vi "Menu Handler.vi"(7 "Sub Panel":refnum<vi>, 8 "error in (no error)":errorcluster, 9 "ItemTag":string, 10 "Menu in":refnum<k9>, 11 "queue out":refnum<queue>) -> (0 "Error Out":errorcluster, 3 "Log 10?":bool=TRUE)   [LabVIEW 2015]
uses:
  Type Defs/OCT Hardware States.ctl
  Classes/DAQ/DAQ Status States.ctl
  Classes/DAQ/DAQ Control Functional Global States.ctl
  Classes/Processing/Filter/Filter List.ctl
  Classes/Processing/Filter/Kernel Size.ctl
  Classes/Processing/Processing.lvclass
  Classes/Processing/Intensity/Intensity Processing.lvclass
  Classes/Processing/Filter/Filter.lvclass
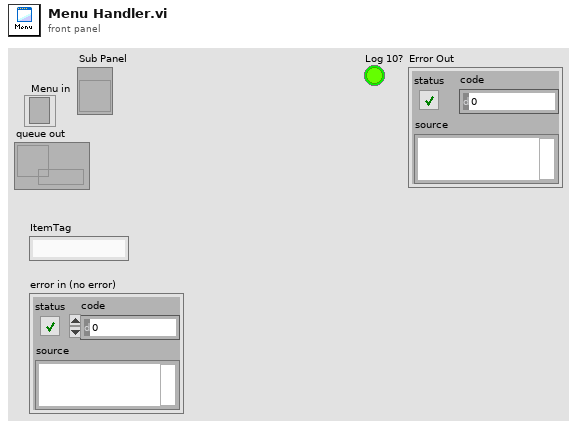
[diagram p1: front panel]
types:
  T1 = typedef "DAQ Status States.ctl" = enum16{"Get", "Show"}
  T2 = typedef "OCT Hardware States.ctl" = enum16{"Acquire Data", "Initialize Laser", "Initialize Galvos", "Startup", "Reset DAQ", "Background Subtraction", "Acquire Background", "Update DAQ Parameters", "Stop", "Set Clock", "Initialize DAQ", "Set Resampling Array", "Save Sweep", "Configure Laser", "128 x 128", "512 x 1", "512 x 512", "Review Data", "Configure Trigger", "Update Galvos", "Update Filter", "Fire Digital Output", "Configure Digital Output", "Save Galvo Settings", "Load Galvo Settings"}
  T3 = typedef "DAQ Control Functional Global States.ctl" = enum16{"Status", "Set Processing Finished", "Reset", "Clear", "Set DAQ Finished"}
  T4 = enum32{"Invalid", "Standard", "Closed", "Hidden", "Minimized", "Maximized"}
  T5 = typedef "Kernel Size.ctl" = enum16{"3x3", "5x5", "3x5", "5x3"}
  T6 = typedef "Filter.lvclass/Filter List.ctl" = enum16{"None", "Std. Dev.", "Speckle Variance"}
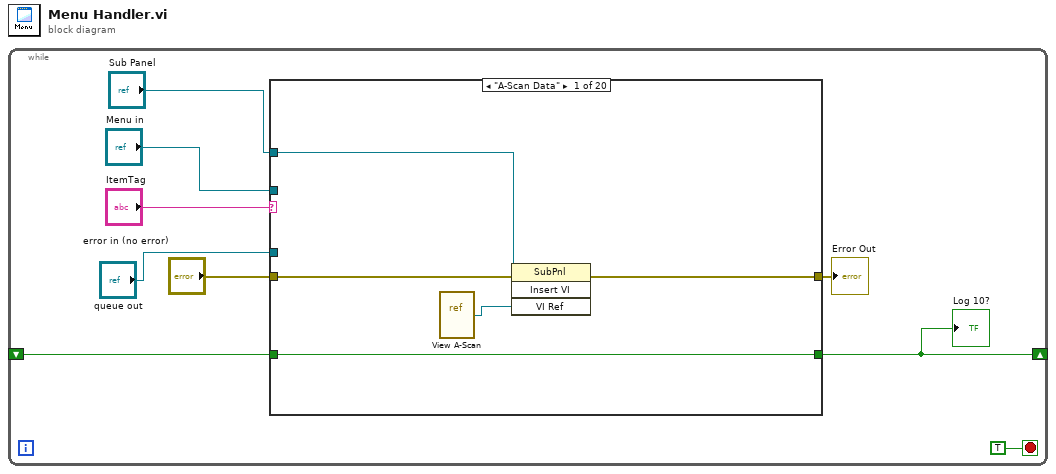
[diagram p0: block diagram]
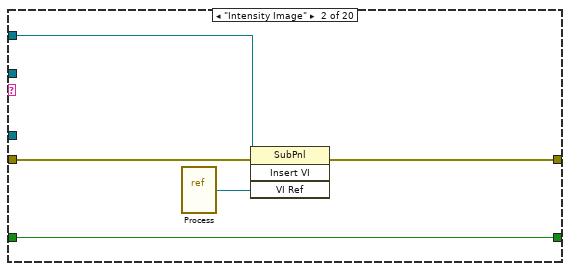
[diagram p2: hidden frame]
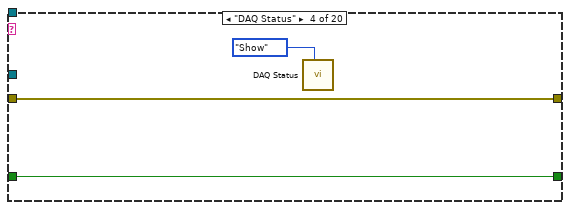
[diagram p4: hidden frame]
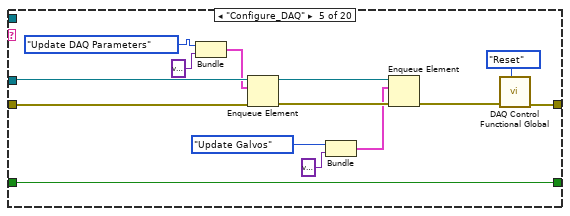
[diagram p5: hidden frame]
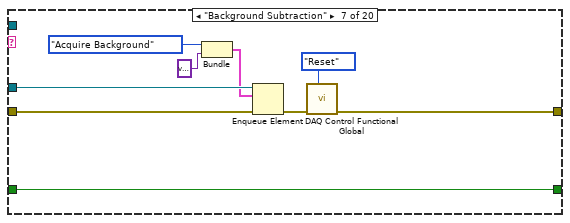
[diagram p7: hidden frame]
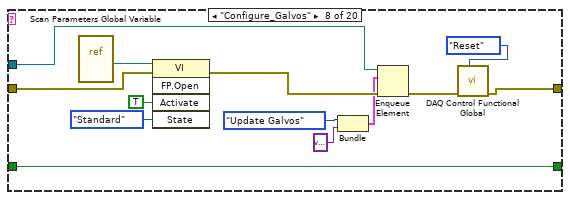
[diagram p8: hidden frame]
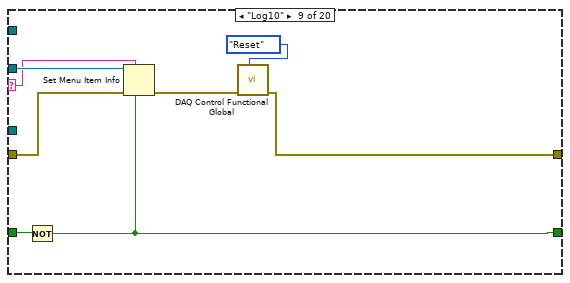
[diagram p9: hidden frame]
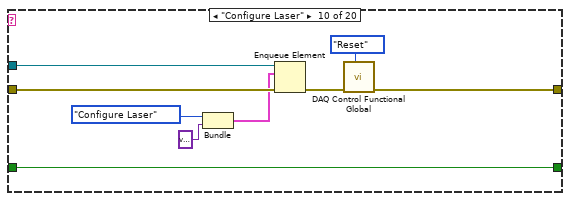
[diagram p10: hidden frame]
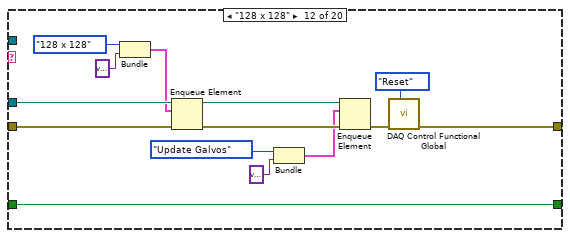
[diagram p12: hidden frame]
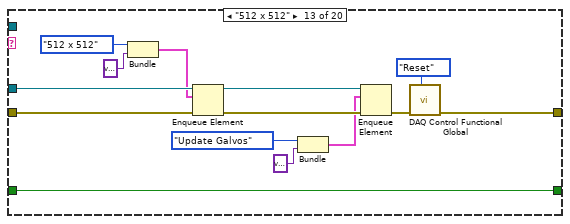
[diagram p13: hidden frame]
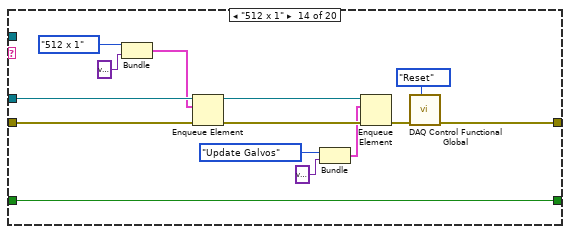
[diagram p14: hidden frame]
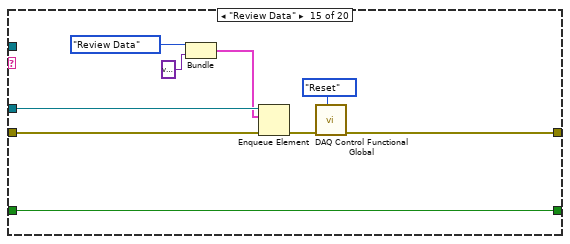
[diagram p15: hidden frame]
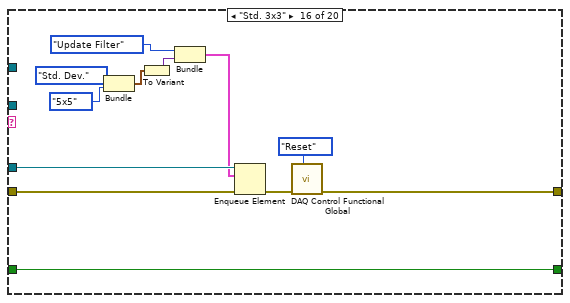
[diagram p16: hidden frame]
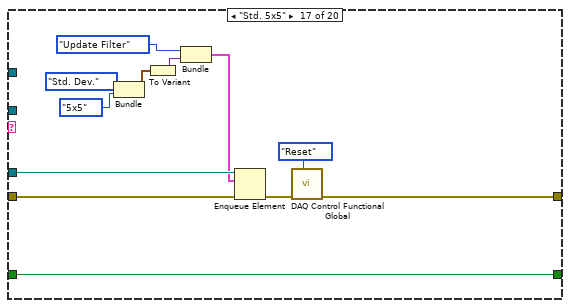
[diagram p17: hidden frame]
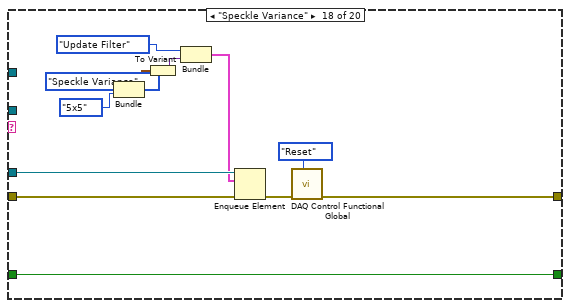
[diagram p18: hidden frame]
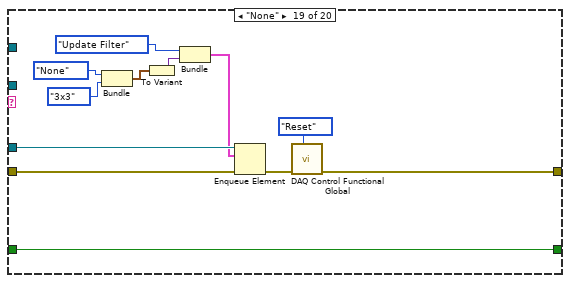
[diagram p19: hidden frame]
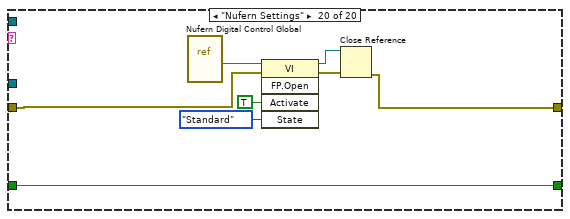
[diagram p20: hidden frame]
diagram:
  n1 = while {
    shift-right: [w2] -> _
    shift-left: _ -> [w3]
    stop <- TRUE stop-if-true
    n2 = case shown="\"A-Scan Data\"" "ItemTag" {
      selector: "ItemTag" -> [_ _ _ _ _ _ _ _ w66 _ _ _ _ _ _ _ _ _ _ _]
      tunnel: "queue out" -> [_ _ _ _ w38 _ w47 w57 _ w79 _ w91 w105 w119 w131 w143 w155 w167 w179 _]
      tunnel: "error in (no error)" -> [w14 w19 w21 w23 w37 w40 w48 w55 w68 w78 w81 w90 w104 w118 w130 w142 w154 w166 w178 w184]
      tunnel: "Menu in" -> [_ _ _ _ _ _ _ _ w70 _ _ _ _ _ _ _ _ _ _ _]
      tunnel: [w13 w18 w21 w23 w32 w40 w45 w54 w67 w75 w81 w89 w103 w117 w128 w140 w152 w164 w176 w182] -> w5
      tunnel: "Sub Panel" -> [w12 w17 _ _ _ _ _ _ _ _ _ _ _ _ _ _ _ _ _ _]
      tunnel: [w10 w15 w20 w22 w31 w39 w44 w53 w64 w74 w80 w88 w102 w116 w127 w139 w151 w163 w175 w188] -> w2
      tunnel: w3 -> [w10 w15 w20 w22 w31 w39 w44 w53 w63 w74 w80 w88 w102 w116 w127 w139 w151 w163 w175 w188]
      frame "A-Scan Data" {
        n3 = vi-ref "View A-Scan.vi"() -> (w11:refnum<vi>)
        n4 = invoke class="SubPnl" method="Insert VI"(reference=w12, error in=w14, "VI Ref"=w11) -> (error out=w13:errorcluster)  [unwired: 1 in, 3 out]
      }
      frame "Intensity Image" {
        n5 = vi-ref "Process.vi"() -> (w16:refnum<vi>)
        n6 = invoke class="SubPnl" method="Insert VI"(reference=w17, error in=w19, "VI Ref"=w16) -> (error out=w18:errorcluster)  [unwired: 1 in, 3 out]
      }
      frame "Nothing", Default {
      }
      frame "DAQ Status" {
        n7 = call "DAQ Status.vi"("Enum"=DAQ_Status_States."Show") -> ()  [unwired: 9 in, 2 out]
      }
      frame "Configure_DAQ" {
        n8 = Bundle("element"=OCT_Hardware_States."Update DAQ Parameters", variant) -> (w28:cluster{"element":T2, variant})  [unwired: 1 in]
        n9 = Enqueue Element(queue=w38, element=w28, error in (no error)=w37) -> (queue out=w34:refnum<queue>, error out=w35:errorcluster)  [unwired: 1 in, 1 out]
        n10 = Bundle("element"=OCT_Hardware_States."Update Galvos", variant) -> (w25:cluster{"element":T2, variant})  [unwired: 1 in]
        n11 = Enqueue Element(queue=w34, element=w25, error in (no error)=w35) -> (error out=w33:errorcluster)  [unwired: 1 in, 2 out]
        n12 = call "DAQ Control Functional Global.vi"("State"=DAQ_Control_Functional_Global_States."Reset", "Error In"=w33) -> ("Error Out"=w32:errorcluster)  [unwired: 6 in, 3 out]
      }
      frame "K-Space Correction" {
      }
      frame "Background Subtraction" {
        n13 = Bundle("element"=OCT_Hardware_States."Acquire Background", variant) -> (w41:cluster{"element":T2, variant})  [unwired: 1 in]
        n14 = Enqueue Element(queue=w47, element=w41, error in (no error)=w48) -> (error out=w46:errorcluster)  [unwired: 1 in, 2 out]
        n15 = call "DAQ Control Functional Global.vi"("State"=DAQ_Control_Functional_Global_States."Reset", "Error In"=w46) -> ("Error Out"=w45:errorcluster)  [unwired: 6 in, 3 out]
      }
      frame "Configure_Galvos" {
        n16 = vi-ref "Scan Parameters Global Variable.vi"() -> (w62:refnum<vi>)
        n17 = invoke class="VI" method="FP.Open"(reference=w62, error in=w55, "Activate"=TRUE ("Activate?"), "State"=T4."Standard") -> (error out=w56:errorcluster)  [unwired: 1 in, 4 out]
        n18 = Bundle("element"=OCT_Hardware_States."Update Galvos", variant) -> (w50:cluster{"element":T2, variant})  [unwired: 1 in]
        n19 = Enqueue Element(queue=w57, element=w50, error in (no error)=w56) -> (error out=w59:errorcluster)  [unwired: 1 in, 2 out]
        n20 = call "DAQ Control Functional Global.vi"("State"=DAQ_Control_Functional_Global_States."Reset", "Error In"=w59) -> ("Error Out"=w54:errorcluster)  [unwired: 6 in, 3 out]
      }
      frame "Log10" {
        n21 = Not(x=w63) -> (.not. x?=w64:bool)
        n22 = Set Menu Item Info(6:w64, 7:w66, 8:w68, 11:w70) -> (0:w65:errorcluster)  [unwired: 3 in, 1 out]
        n23 = call "DAQ Control Functional Global.vi"("State"=DAQ_Control_Functional_Global_States."Reset", "Error In"=w65) -> ("Error Out"=w67:errorcluster)  [unwired: 6 in, 3 out]
      }
      frame "Configure Laser" {
        n24 = Bundle("element"=OCT_Hardware_States."Configure Laser", variant) -> (w71:cluster{"element":T2, variant})  [unwired: 1 in]
        n25 = Enqueue Element(queue=w79, element=w71, error in (no error)=w78) -> (error out=w76:errorcluster)  [unwired: 1 in, 2 out]
        n26 = call "DAQ Control Functional Global.vi"("State"=DAQ_Control_Functional_Global_States."Reset", "Error In"=w76) -> ("Error Out"=w75:errorcluster)  [unwired: 6 in, 3 out]
      }
      frame "Laser Status" {
      }
      frame "128 x 128" {
        n27 = Bundle("element"=OCT_Hardware_States."128 x 128", variant) -> (w86:cluster{"element":T2, variant})  [unwired: 1 in]
        n28 = Enqueue Element(queue=w91, element=w86, error in (no error)=w90) -> (queue out=w93:refnum<queue>, error out=w94:errorcluster)  [unwired: 1 in, 1 out]
        n29 = Bundle("element"=OCT_Hardware_States."Update Galvos", variant) -> (w82:cluster{"element":T2, variant})  [unwired: 1 in]
        n30 = Enqueue Element(queue=w93, element=w82, error in (no error)=w94) -> (error out=w92:errorcluster)  [unwired: 1 in, 2 out]
        n31 = call "DAQ Control Functional Global.vi"("State"=DAQ_Control_Functional_Global_States."Reset", "Error In"=w92) -> ("Error Out"=w89:errorcluster)  [unwired: 6 in, 3 out]
      }
      frame "512 x 512" {
        n32 = Bundle("element"=OCT_Hardware_States."512 x 512", variant) -> (w99:cluster{"element":T2, variant})  [unwired: 1 in]
        n33 = Enqueue Element(queue=w105, element=w99, error in (no error)=w104) -> (queue out=w107:refnum<queue>, error out=w108:errorcluster)  [unwired: 1 in, 1 out]
        n34 = Bundle("element"=OCT_Hardware_States."Update Galvos", variant) -> (w96:cluster{"element":T2, variant})  [unwired: 1 in]
        n35 = Enqueue Element(queue=w107, element=w96, error in (no error)=w108) -> (error out=w106:errorcluster)  [unwired: 1 in, 2 out]
        n36 = call "DAQ Control Functional Global.vi"("State"=DAQ_Control_Functional_Global_States."Reset", "Error In"=w106) -> ("Error Out"=w103:errorcluster)  [unwired: 6 in, 3 out]
      }
      frame "512 x 1" {
        n37 = Bundle("element"=OCT_Hardware_States."512 x 1", variant) -> (w113:cluster{"element":T2, variant})  [unwired: 1 in]
        n38 = Enqueue Element(queue=w119, element=w113, error in (no error)=w118) -> (queue out=w121:refnum<queue>, error out=w122:errorcluster)  [unwired: 1 in, 1 out]
        n39 = Bundle("element"=OCT_Hardware_States."Update Galvos", variant) -> (w110:cluster{"element":T2, variant})  [unwired: 1 in]
        n40 = Enqueue Element(queue=w121, element=w110, error in (no error)=w122) -> (error out=w120:errorcluster)  [unwired: 1 in, 2 out]
        n41 = call "DAQ Control Functional Global.vi"("State"=DAQ_Control_Functional_Global_States."Reset", "Error In"=w120) -> ("Error Out"=w117:errorcluster)  [unwired: 6 in, 3 out]
      }
      frame "Review Data" {
        n42 = Bundle("element"=OCT_Hardware_States."Review Data", variant) -> (w124:cluster{"element":T2, variant})  [unwired: 1 in]
        n43 = Enqueue Element(queue=w131, element=w124, error in (no error)=w130) -> (error out=w129:errorcluster)  [unwired: 1 in, 2 out]
        n44 = call "DAQ Control Functional Global.vi"("State"=DAQ_Control_Functional_Global_States."Reset", "Error In"=w129) -> ("Error Out"=w128:errorcluster)  [unwired: 6 in, 3 out]
      }
      frame "Std. 3x3" {
        n45 = Bundle("Filter"=Filter_List."Std. Dev.", "Kernel Size"=Kernel_Size."5x5") -> (w133:cluster{"Filter":T6, "Kernel Size":T5})  [unwired: 1 in]
        n46 = To Variant(anything=w133) -> (Variant=w136:variant)
        n47 = Bundle("element"=OCT_Hardware_States."Update Filter", "Variant"=w136) -> (w137:cluster{"element":T2, "Variant":variant})  [unwired: 1 in]
        n48 = Enqueue Element(queue=w143, element=w137, error in (no error)=w142) -> (error out=w141:errorcluster)  [unwired: 1 in, 2 out]
        n49 = call "DAQ Control Functional Global.vi"("State"=DAQ_Control_Functional_Global_States."Reset", "Error In"=w141) -> ("Error Out"=w140:errorcluster)  [unwired: 6 in, 3 out]
      }
      frame "Std. 5x5" {
        n50 = Bundle("Filter"=Filter_List."Std. Dev.", "Kernel Size"=Kernel_Size."5x5") -> (w145:cluster{"Filter":T6, "Kernel Size":T5})  [unwired: 1 in]
        n51 = To Variant(anything=w145) -> (Variant=w148:variant)
        n52 = Bundle("element"=OCT_Hardware_States."Update Filter", "Variant"=w148) -> (w149:cluster{"element":T2, "Variant":variant})  [unwired: 1 in]
        n53 = Enqueue Element(queue=w155, element=w149, error in (no error)=w154) -> (error out=w153:errorcluster)  [unwired: 1 in, 2 out]
        n54 = call "DAQ Control Functional Global.vi"("State"=DAQ_Control_Functional_Global_States."Reset", "Error In"=w153) -> ("Error Out"=w152:errorcluster)  [unwired: 6 in, 3 out]
      }
      frame "Speckle Variance" {
        n55 = Bundle("Filter"=Filter_List."Speckle Variance", "Kernel Size"=Kernel_Size."5x5") -> (w157:cluster{"Filter":T6, "Kernel Size":T5})  [unwired: 1 in]
        n56 = To Variant(anything=w157) -> (Variant=w160:variant)
        n57 = Bundle("element"=OCT_Hardware_States."Update Filter", "Variant"=w160) -> (w161:cluster{"element":T2, "Variant":variant})  [unwired: 1 in]
        n58 = Enqueue Element(queue=w167, element=w161, error in (no error)=w166) -> (error out=w165:errorcluster)  [unwired: 1 in, 2 out]
        n59 = call "DAQ Control Functional Global.vi"("State"=DAQ_Control_Functional_Global_States."Reset", "Error In"=w165) -> ("Error Out"=w164:errorcluster)  [unwired: 6 in, 3 out]
      }
      frame "None" {
        n60 = Bundle("Filter"=Filter_List."None", "Kernel Size"=Kernel_Size."3x3") -> (w169:cluster{"Filter":T6, "Kernel Size":T5})  [unwired: 1 in]
        n61 = To Variant(anything=w169) -> (Variant=w172:variant)
        n62 = Bundle("element"=OCT_Hardware_States."Update Filter", "Variant"=w172) -> (w173:cluster{"element":T2, "Variant":variant})  [unwired: 1 in]
        n63 = Enqueue Element(queue=w179, element=w173, error in (no error)=w178) -> (error out=w177:errorcluster)  [unwired: 1 in, 2 out]
        n64 = call "DAQ Control Functional Global.vi"("State"=DAQ_Control_Functional_Global_States."Reset", "Error In"=w177) -> ("Error Out"=w176:errorcluster)  [unwired: 6 in, 3 out]
      }
      frame "Nufern Settings" {
        n65 = vi-ref "Nufern Digital Control Global.vi"() -> (w187:refnum<vi>)
        n66 = invoke class="VI" method="FP.Open"(reference=w187, error in=w184, "Activate"=TRUE ("Activate?"), "State"=T4."Standard") -> (reference out=w181:refnum<vi>, error out=w183:errorcluster)  [unwired: 1 in, 3 out]
        n67 = Close Reference(reference=w181, error in (no error)=w183) -> (error out=w182:errorcluster)
      }
    }
    "Error Out" <- w5
    "Log 10?" <- w2
  }
